vi "quatMultiply.vi"(10 "q2":dbl[](array[numeric])=[4.0, 5.0, 6.0, 7.0], 11 "q1":dbl[](array[numeric])=[1.0, 12.0, 3.0, 4.0]) -> (3 "qResult":dbl[](array[numeric]))   [LabVIEW 2020]
uses:
  <vilib>/imath/engines/lvmath2/RunTimeEngine/IndexRead/NIMS V(S).vi
  <instcachedir>/0/NIMS V(S)_0488751826AF41519A22953C041130DC.lvgen/NIMS V(S)_0488751826AF41519A22953C041130DC_000.vi
  <vilib>/imathl/engines/lvmath/Functions/Error Handling/Create Error.vi
  <vilib>/imath/engines/lvmath2/RunTimeEngine/NodeEndStatement/NIMS_NodeEndStatement_Output.vi
  <instcachedir>/0/NIMS_NodeEndStatement_Output_53EC0D466D134D7ABD903AC30B43404B.lvgen/NIMS_NodeEndStatement_Output_53EC0D466D134D7ABD903AC30B43404B_005.vi
  <vilib>/imath/engines/lvmath2/RunTimeEngine/ErrorHandling/NIMS_Finalize Error.vi
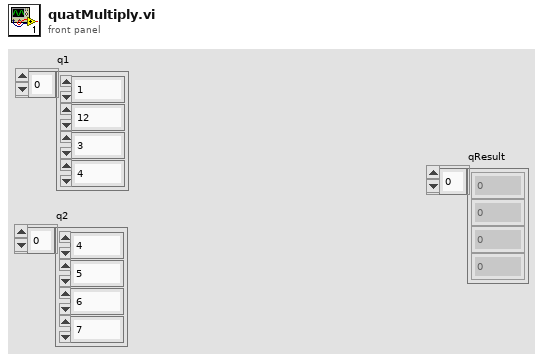
[diagram p1: front panel]
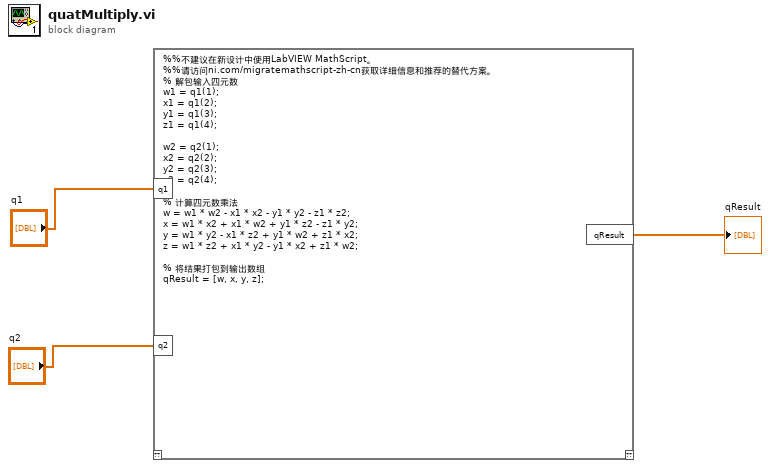
[diagram p0: block diagram]
diagram:
  n1 = mathscript code="%%不建议在新设计中使用LabVIEW MathScript。\n%%请访问ni.com/migratemathscript-zh-cn获取详细信息和推荐的替代方案。\n% 解包输入四元数\nw1 = q1(1);\nx1 = q1(2);\ny1 = q1(3);\nz1 = q1(4);\n\nw2 = q2(1);\nx2 = q2(2);\ny2 = q2(3);\nz2 = q2(4);\n\n% 计算四元数乘法\nw = w1 * w2 - x1 * x2 - y1 * y2 - z1 * z2;\nx = w1 * x2 + x1 * w2 + y1 * z2 - z1 * y2;\ny = w1 * y2 - x1 * z2 + y1 * w2 + z1 * x2;\nz = w1 * z2 + x1 * y2 - y1 * x2 + z1 * w2;\n\n% 将结果打包到输出数组\nqResult = [w, x, y, z];"("q1"="q1", "q2"="q2") -> ("qResult"=→"qResult":dbl[])  [unwired: 1 in, 1 out]
